vi "Exp3_SCADA.vi"() -> ()   [LabVIEW 2025]
panel:
  out "Waveform Chart":i32(graph)
  out "Numeric":dbl
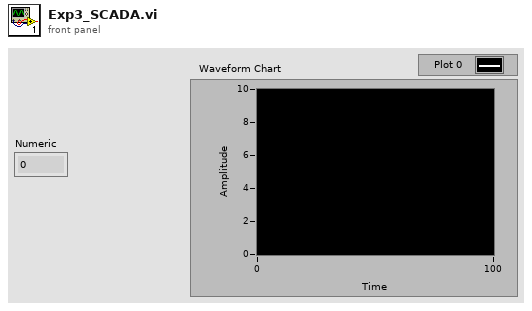
[diagram p1: front panel]
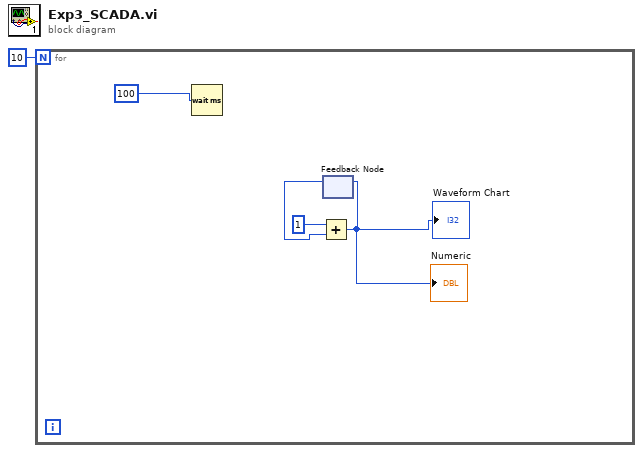
[diagram p0: block diagram]
diagram:
  n1 = for {
    N: 10 -> [_]
    n2 = Wait (ms)(milliseconds to wait=100) -> ()  [unwired: 1 out]
    n3 = feedback #1() -> (w3:i32)  [unwired: 1 in]
    n4 = Add(x=1, y=w3) -> (x+y=w2:i32)
    "Numeric" <- w2
    "Waveform Chart" <- w2
    n5 = feedback-in #1(w2) -> ()
  }
